vi "logoutSession.vi"(8 "error in (no error)":errorcluster, 11 "SM1000-control in":T1) -> (0 "error out":errorcluster, 3 "SM1000-control out":T1)   [LabVIEW 2013, in "HardwareCharacterization.lvlib" / "HC-SM1000.lvclass"]
doc: "Disconnect an EC device session.\n\nWhen session communication is completed, the client closes the session via a call to this method. Once the session is closed, another new session may be opened to the same or other EC1000 devices via a call to 'loginSession'.\nNote that if a job was streamed out to the EC1000 and was still executing when the logout was invoked, the job will be immediately aborted."
uses:
  HC-SM1000.lvclass
  Object-reference.ctl
  HC-SM1000.lvclass/HC-SM1000.ctl
  Custom-errors.ctl
  C:/Users/vangeste/Desktop/2015-05-29 - SLM - MAIF/HC-HardwareCharacterization/Sources/SM1000/LECSession.dll
  LECSession.dll
  DOTNET-error-int.vi
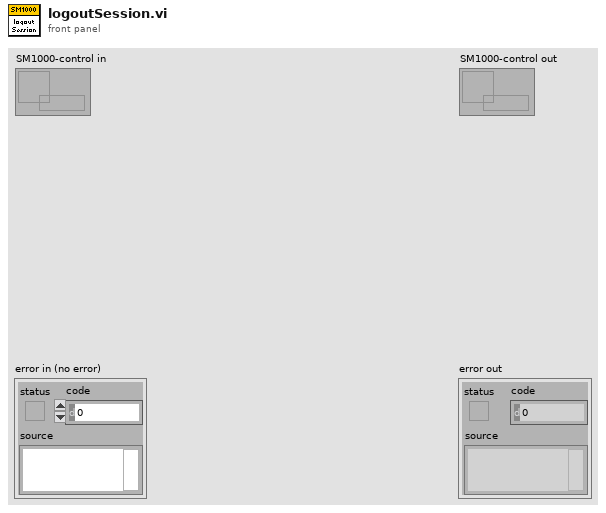
[diagram p1: front panel]
types:
  T1 = typedef "HardwareCharacterization.lvlib/HC-SM1000.lvclass/Object-reference.ctl" = refnum<data-value>
  T2 = typedef "HardwareCharacterization.lvlib/HC-SM1000.lvclass/Custom-errors.ctl" = enum16{"No error", "Not implemented", "Command not recognized", "Invalid input", "No connection", "Timeout", "Resource not loaded"}
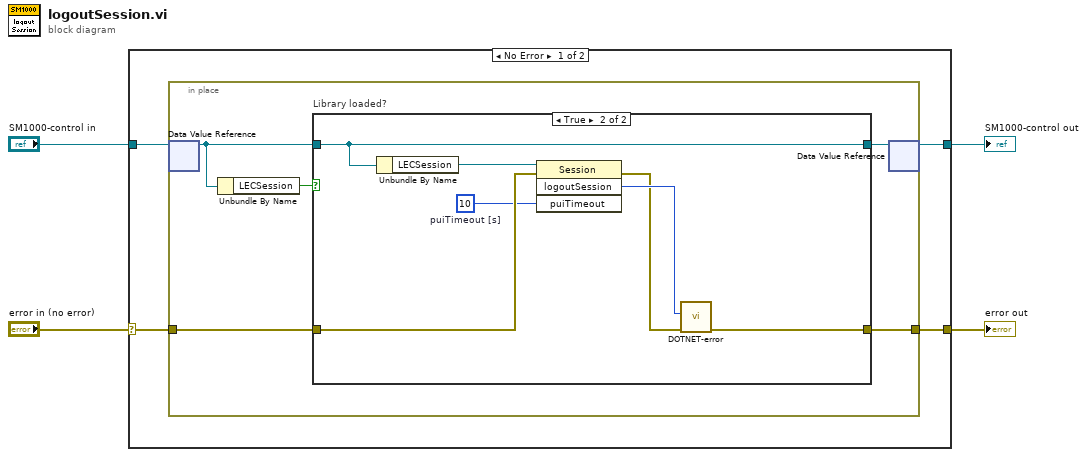
[diagram p0: block diagram]
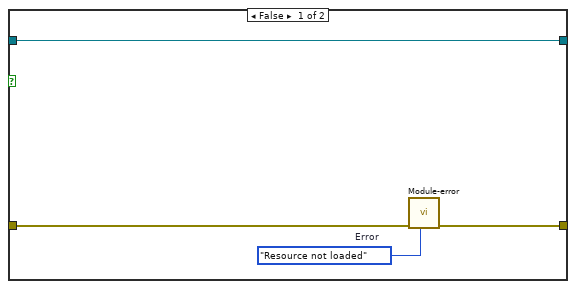
[diagram p2: hidden frame]
diagram:
  n1 = case shown="No Error" "error in (no error)" {
    selector: "error in (no error)" -> [w6 w26]
    tunnel: [w5 w26] -> w3
    tunnel: [w7 w25] -> w1
    tunnel: "SM1000-control in" -> [w8 w25]
    frame No Error {
      n2 = in-place {
        in-place-border: w6 -> [w13]
        in-place-border: [w10] -> w5
        n3 = in-place-dvr #1(w8) -> (w11:refnum<class "HC-SM1000.lvclass">)  [unwired: 1 out]
        n4 = Unbundle By Name(w11) -> ("LECSession"=w12:bool)
        n5 = case "Library loaded?" shown="True" w12 {
          tunnel: w13 -> [w17 w23]
          tunnel: w11 -> [w15 w22]
          tunnel: [w16 w20] -> w10
          tunnel: [w15 w22] -> w9
          frame False {
            w14 = Custom-errors."Resource not loaded"  # Error
            n6 = call "Module-error.vi"("Error"=w14, "error in (no error)"=w17) -> ("error out"=w16:errorcluster)  [unwired: 9 in]
          }
          frame True {
            w21 = u32 10  # puiTimeout [s]
            n7 = Unbundle By Name(w22) -> ("LECSession"=w24:refnum<k24>)
            n8 = invoke class="Session" method="logoutSession"(reference=w24, error in=w23, "puiTimeout"=w21) -> (error out=w18:errorcluster, "logoutSession"=w19:u32)  [unwired: 1 in, 2 out]
            n9 = call-poly "DOTNET-error.vi"("error in (no error)"=w18, "Retun code"=w19) -> ("error out"=w20:errorcluster)  [unwired: 9 in]
          }
        }
        n10 = in-place-dvr #1(w9) -> (w7:T1)  [unwired: 1 out]
      }
    }
    frame Error {
    }
  }
  "error out" <- w3
  "SM1000-control out" <- w1
